vi "Connect.vi"(8 "error in (no error)":errorcluster, 10 "Port (8125)":u16=8125, 11 "Host Name (localhost)":string="localhost") -> (0 "error out":errorcluster, 3 "StatD Interface out":refnum<class "StatD Interface.lvclass">)   [LabVIEW 2011, in "StatD Interface.lvclass"]
doc: "Creates the StatD Interface and prepares the connection for use."
uses:
  StatD Interface.lvclass
  StatD Interface.lvclass/StatD Interface.ctl
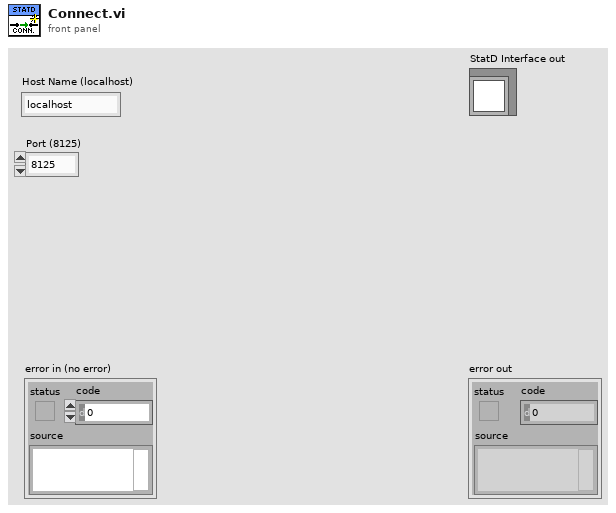
[diagram p1: front panel]
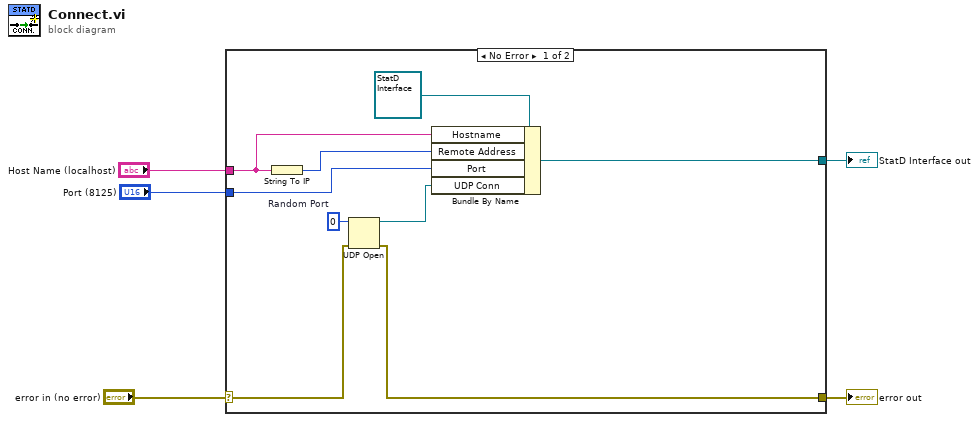
[diagram p0: block diagram]
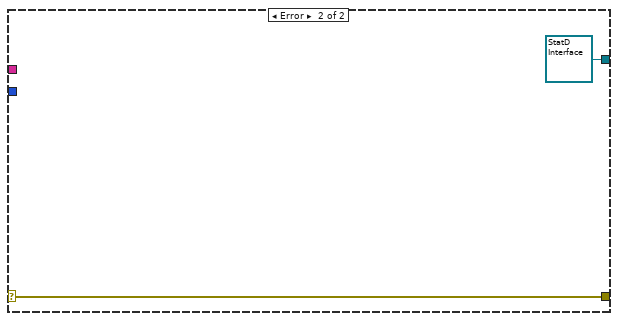
[diagram p2: hidden frame]
diagram:
  n1 = case shown="No Error" "error in (no error)" {
    selector: "error in (no error)" -> [w14 w16]
    tunnel: [w7 w16] -> w4
    tunnel: "Host Name (localhost)" -> [w12 _]
    tunnel: "Port (8125)" -> [w10 _]
    tunnel: [w6 refnum<class "StatD Interface.lvclass"> refnum ("StatD Interface out")] -> w1
    frame No Error {
      w8 = u16 0  # Random Port
      n2 = String To IP(1:w12) -> (0:w11:u32)
      n3 = UDP Open(8:w14, 11:w8) -> (port=w9:refnum<k16>, 0:w7:errorcluster)  [unwired: 3 in, 1 out]
      n4 = Bundle By Name(cluster=refnum<class "StatD Interface.lvclass"> refnum ("StatD Interface out"), "Hostname"=w12, "Remote Address"=w11, "Port"=w10, "UDP Conn"=w9) -> (w6:refnum<class "StatD Interface.lvclass">)
    }
    frame Error {
    }
  }
  "error out" <- w4
  "StatD Interface out" <- w1
